vi "Terranova908A_remote.vi"() -> ()   [LabVIEW 2009]
uses:
  <vilib>/Instr/_visa.llb/VISA Configure Serial Port (Instr).vi
panel:
  out "Boolean":bool
  out "read buffer Main":string
  in  "stop":bool
  out "Gas2":dbl caption="torr" format="%_3f"
  out "Gas1":dbl caption="torr" format="%_3f"
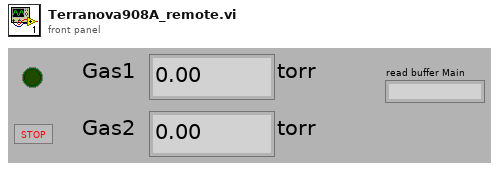
[diagram p1: front panel]
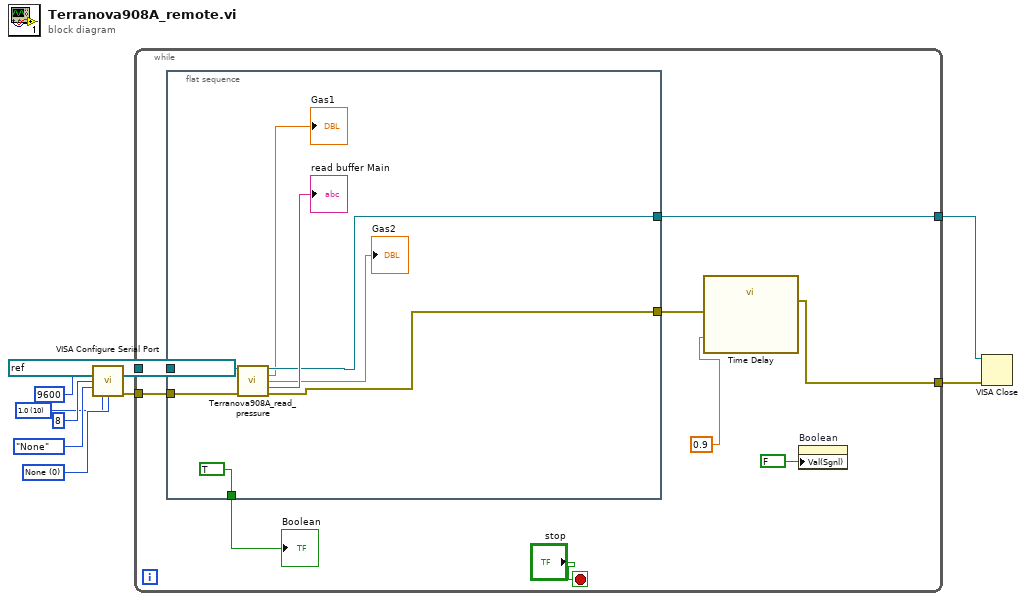
[diagram p0: block diagram]
diagram:
  w2 = u16 10 items=["1.0"=10, "1.5"=15, "2.0"=20] ("stop bits (10: 1 bit)")
  w6 = u16 0 items=["None", "XON/XOFF", "RTS/CTS", "XON/XOFF & RTS/CTS", "DTR/DSR", "XON/XOFF & DTR/DSR"] ("flow control (0:none)")
  n1 = call-poly "VISA Configure Serial Port"("VISA resource name"=refnum<visa-resource-name> "visa://s132pc1.slac.stanford.edu/COM10", "baud rate (9600)"=u32 9600, "data bits (8)"=u16 8, "parity (0:none)"=enum16{"None", "Odd", "Even", "Mark", "Space"}."None", "stop bits (10: 1 bit)"=w2, "flow control (0:none)"=w6) -> ("VISA resource name out"=w5:refnum<visa-resource-name>, "error out"=w4:errorcluster)  [unwired: 8 in]
  n2 = while {
    tunnel: w5 -> [w19]
    tunnel: w4 -> [w18]
    tunnel: [w17] -> w1
    tunnel: [w13] -> w3
    stop <- "stop" stop-if-true
    n3 = flat-sequence {
      tunnel: w19 -> [w27]
      tunnel: w18 -> [w26]
      tunnel: [w22] -> w17
      tunnel: [w23] -> w12
      tunnel: [TRUE ("Boolean")] -> w11
      frame #0 {
        n4 = call "Terranova908A_read_pressure.vi"("VISA resource name"=w27, "error in (no error)"=w26) -> ("VISA resource name out"=w22:refnum<visa-resource-name>, "pressure"=→"Gas1":dbl, "pressure 2"=→"Gas2":dbl, "read buffer"=→"read buffer Main":string, "error out"=w23:errorcluster)  [unwired: 9 in]
      }
    }
    n5 = call "Time Delay"("error in (no error)"=w12, "Delay Time (s)"=0.9) -> ("error out"=w13:errorcluster)  [unwired: 9 in]
    n6 = property on="Boolean" class="Bool (strict)"("Val(Sgnl)"=FALSE ("Boolean")) -> ()  [unwired: 2 in, 2 out]
    "Boolean" <- w11
  }
  n7 = VISA Close(VISA resource name=w1, error in (no error)=w3) -> ()  [unwired: 1 out]
